vi "mes配置前验证.vi"() -> (0 "管理员":bool, 2 "Success?":bool)   [LabVIEW 2020]
panel:
  in  "登录":bool
  in  "注销":bool
  in  "Password":string caption="密   码:"
  in  "UserName":string caption="用户名:"
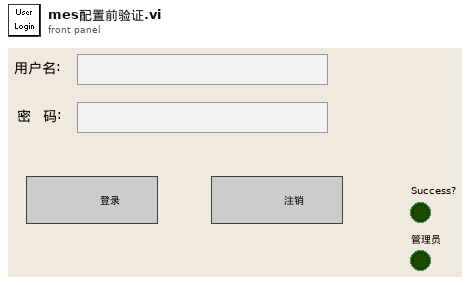
[diagram p1: front panel]
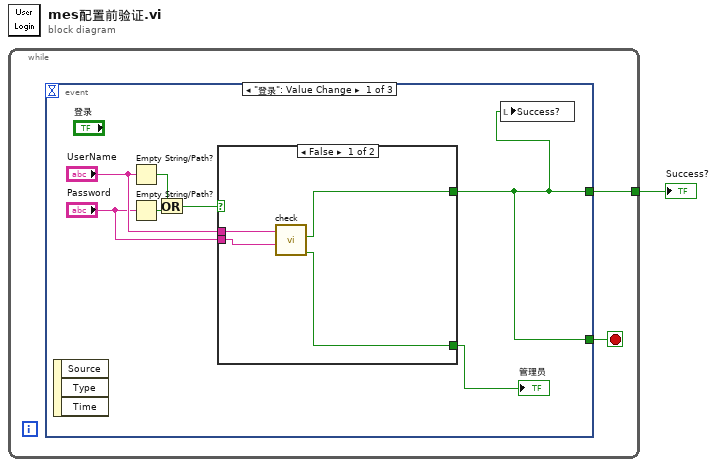
[diagram p0: block diagram]
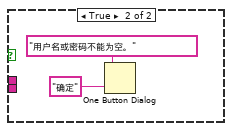
[diagram p2: hidden frame]
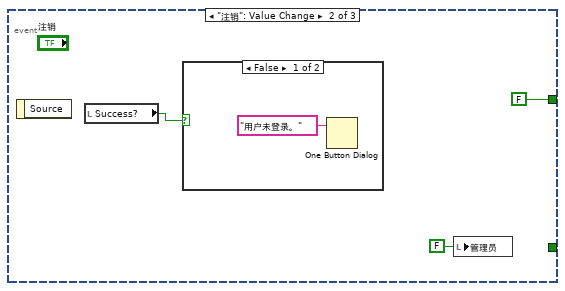
[diagram p3: hidden frame]
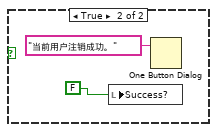
[diagram p4: hidden frame]
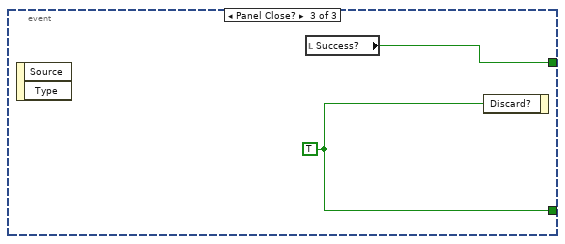
[diagram p5: hidden frame]
diagram:
  n1 = while {
    tunnel: [w2] -> w1
    stop <- w3 stop-if-true
    n2 = event shown="[0] \"登录\": Value Change" {
      selector: _ -> [_ _ _]
      dyn-events: _ -> [_ _ _]
      timeout: _ -> [_ _ _]
      tunnel: [w4 _ w24] -> w3
      tunnel: [w4 FALSE ("Success?") w23] -> w2
      event "登录": Value Change {
        n3 = event-data() -> ()  [unwired: 1 in, 3 out]
        n4 = Empty String/Path?(string/path="UserName") -> (empty?=w9:bool)
        n5 = Empty String/Path?(string/path="Password") -> (empty?=w10:bool)
        n6 = Or(x=w9, y=w10) -> (x .or. y?=w8:bool)
        n7 = case shown="False" w8 {
          tunnel: "UserName" -> [w14 _]
          tunnel: "Password" -> [w13 _]
          tunnel: [w12 _] -> w4
          tunnel: [w11 _] -> w5
          frame False {
            n8 = call "check.vi"("Password"=w13, "UserName"=w14) -> ("管理员"=w11:bool, "Success?"=w12:bool)  [unwired: 8 in]
          }
          frame True {
            n9 = One Button Dialog(message="用户名或密码不能为空。", button name ("OK")="确定") -> ()  [unwired: 1 out]
          }
        }
        "管理员" <- w5
        n10 = local write "Success?"(w4) -> ()
      }
      event "注销": Value Change {
        n11 = event-data() -> ()  [unwired: 1 in, 1 out]
        n12 = local read "Success?"() -> (w18:bool)
        n13 = case shown="False" w18 {
          frame False {
            n14 = One Button Dialog(message="用户未登录。" ("消息")) -> ()  [unwired: 1 in, 1 out]
          }
          frame True {
            n15 = local write "Success?"(FALSE ("Success?")) -> ()
            n16 = One Button Dialog(message="当前用户注销成功。" ("消息")) -> ()  [unwired: 1 in, 1 out]
          }
        }
        n17 = local write "管理员"(FALSE ("管理员")) -> ()
      }
      event Panel Close? {
        w24 = TRUE
        n18 = event-data() -> ()  [unwired: 1 in, 2 out]
        n19 = local read "Success?"() -> (w23:bool)
        n20 = event-data("Discard?"=w24) -> ()  [unwired: 1 in, 1 out]
      }
    }
  }
  "Success?" <- w1
